vi "homersekletmasodik.vi"() -> ()   [LabVIEW 2011]
panel:
  out "Hõmérsékletek":cluster{dbl, "hõmérséklet":dbl}(graph)
  out "String":string
  in  "min":dbl
  in  "max":dbl
  in  "hõmérséklet":dbl(slide) scale=0.0..10.0
  in  "stop":bool
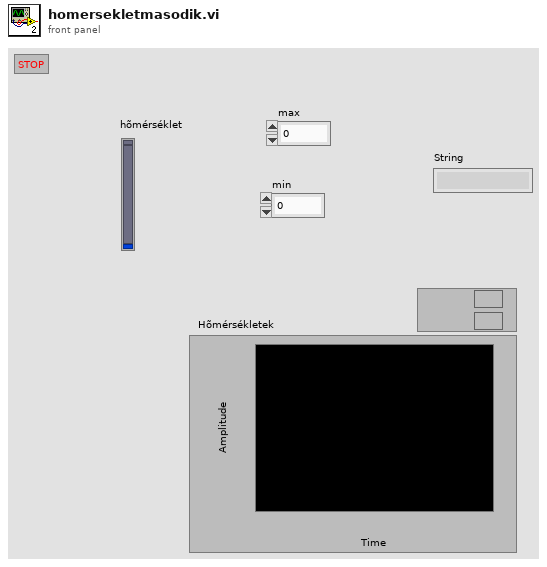
[diagram p1: front panel]
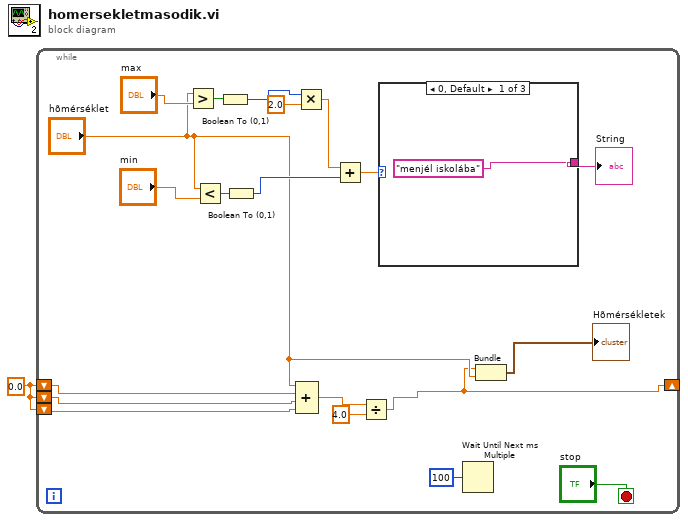
[diagram p0: block diagram]
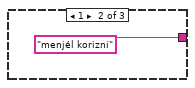
[diagram p2: hidden frame]
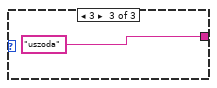
[diagram p3: hidden frame]
diagram:
  w1 = 0.0
  n1 = while {
    shift-right: [w2] -> _
    shift-left: w1 -> [w5]
    shift-left: w1 -> [w4]
    shift-left: w1 -> [w3]
    stop <- "stop" stop-if-true
    n2 = Greater?(x="hõmérséklet", y="max") -> (0:w16:bool)
    n3 = Less?(x="hõmérséklet", y="min") -> (x < y?=w15:bool)
    n4 = Boolean To (0,1)(Boolean=w16) -> (0, 1=w13:i16)
    n5 = Boolean To (0,1)(Boolean=w15) -> (0, 1=w12:i16)
    n6 = Multiply(x=w13, y=2.0) -> (x*y=w11:dbl)
    n7 = Compound Arithmetic op=ADD("hõmérséklet", w5, w4, w3) -> (w7:dbl)
    n8 = Add(x=w11, y=w12) -> (x+y=w19:dbl)
    n9 = Divide(x=w7, y=4.0) -> (x/y=w2:dbl)
    n10 = case shown="0, Default" w19 {
      tunnel: ["menjél iskolába" "menjél korizni" "uszoda"] -> w20
      frame 0, Default {
      }
      frame 1 {
      }
      frame 3 {
      }
    }
    "String" <- w20
    n11 = Wait Until Next ms Multiple(millisecond multiple=u32 100) -> ()  [unwired: 1 out]
    n12 = Bundle(w2, "hõmérséklet"="hõmérséklet") -> (→"Hõmérsékletek":cluster{dbl, "hõmérséklet":dbl})  [unwired: 1 in]
  }
